vi "WPI_AccelerometerADXL362_SPI_Open.vi"(7 "SPI Bus":T1=enum."Invalid", 8 "error in":errorcluster, 9 "Accel Range":T2 items=["+/- 2 g", "+/- 4 g", "+/- 8 g"], 10 "ADXL345 Axes":T3={"X-Axis"=TRUE, "Y-Axis"=FALSE, "Z-Axis"=FALSE}) -> (0 "error out":errorcluster, 3 "AccelerometerDevRef":T4={"DevStatus"={"status"=FALSE, "code"=0, "source"=""}, "Scaling"={"Gain (VoltsPerG)"=0.0, "Center Voltage"=0.0}, "Analog Channels"={"X-Axis"=enum."Invalid", "Y-Axis"=enum."Invalid", "Z-Axis"=enum."Invalid"}, "I2C Bus"=enum."Invalid", "SPI Bus"=enum."Invalid", "Accel Range"=0, "ADXL Axes"={"X-Axis"=FALSE, "Y-Axis"=FALSE, "Z-Axis"=FALSE}, "Handle"=0, "Device Address"=0, "Accel Type"=enum."Analog"} {"Device Address" format="%.0x"; "Accel Range" items=["+/- 2 g", "+/- 4 g", "+/- 8 g", "+/- 16 g"]})   [LabVIEW 2017]
doc: "Opens a reference to the accelerometer you specify. You must open a reference before using any other VIs on this palette.\n\nThis software is licensed. Open the labview\\readme\\WPI Robotics Library Open Source License.txt file for more information."
uses:
  <vilib>/Rock Robotics/WPI/Accelerometer/WPI_AccelerometerDevRef.ctl
  <vilib>/Rock Robotics/WPI/Accelerometer/WPI_AccelerometerScaling.ctl
  <vilib>/Rock Robotics/WPI/Accelerometer/WPI_AccelerometerAnalogChannels.ctl
  <vilib>/Rock Robotics/SystemInterfaces/AI/FPGA_AIChannel.ctl
  <vilib>/Rock Robotics/SystemInterfaces/i2clib/i2c_bus.ctl
  <vilib>/Rock Robotics/SystemInterfaces/spilib/spi_bus.ctl
  <vilib>/Rock Robotics/WPI/Accelerometer/ADXL345 Range.ctl
  <vilib>/Rock Robotics/WPI/Accelerometer/WPI_AccelerometerADXL345 Axes.ctl
  <vilib>/Rock Robotics/WPI/Accelerometer/ADXL362 Range.ctl
  <vilib>/Rock Robotics/SystemInterfaces/NetworkCommunication/NetComm_UsageReport_ResourceType.ctl
  <vilib>/Rock Robotics/WPI/SPI/WPI_SPIMode.ctl
panel:
  # "ADXL"
  # "Analog"
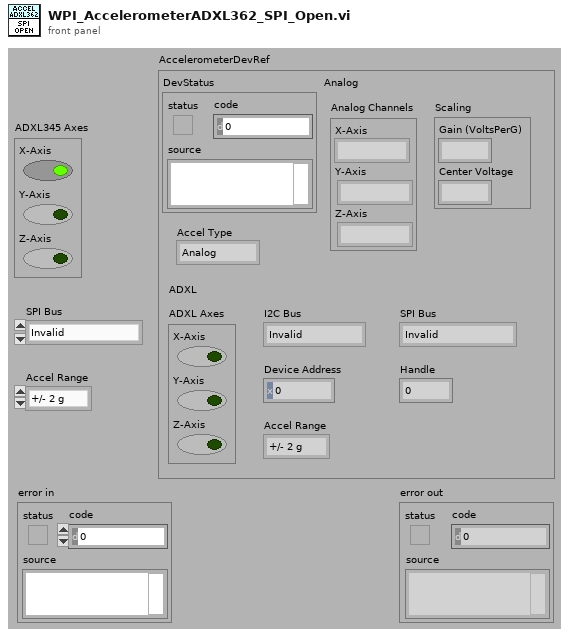
[diagram p1: front panel]
types:
  T1 = typedef "spi_bus.ctl" = enum16{"SPI On-Board, CS0", "SPI On-Board, CS1", "SPI On-Board, CS2", "SPI On-Board, CS3", "SPI MXP", "Invalid"}
  T2 = typedef "ADXL362 Range.ctl" = u8
  T3 = typedef "WPI_AccelerometerADXL345 Axes.ctl" = cluster{"X-Axis":bool, "Y-Axis":bool, "Z-Axis":bool}
  T4 = typedef "WPI_AccelerometerDevRef.ctl" = cluster{"DevStatus":errorcluster, "Scaling":T5, "Analog Channels":T6, "I2C Bus":T8, "SPI Bus":T1, "Accel Range":T9, "ADXL Axes":T3, "Handle":i32, "Device Address":u8, "Accel Type":enum16{"Analog", "ADXL345 I2C", "ADXL345 SPI", "Internal", "ADXL362 SPI"}}
  T5 = typedef "WPI_AccelerometerScaling.ctl" = cluster{"Gain (VoltsPerG)":dbl, "Center Voltage":dbl}
  T6 = typedef "WPI_AccelerometerAnalogChannels.ctl" = cluster{"X-Axis":T7, "Y-Axis":T7, "Z-Axis":T7}
  T7 = typedef "FPGA_AIChannel.ctl" = enum8{"AI 0", "AI 1", "AI 2", "AI 3", "AI MXP 0", "AI MXP 1", "AI MXP 2", "AI MXP 3", "Invalid"}
  T8 = typedef "i2c_bus.ctl" = enum16{"I2C On-Board", "I2C MXP", "Invalid"}
  T9 = typedef "ADXL345 Range.ctl" = u8
  T10 = typedef "WPI_SPIMode.ctl" = enum16{"Mode 0 (Clk Idle Low,Sample on Leading)", "Mode 1 (Clk Idle Low,Sample on Trailing)", "Mode 2 (Clk Idle High,Sample on Leading)", "Mode 3 (Clk Idle High,Sample on Trailing)"}
  T11 = typedef "NetComm_UsageReport_ResourceType.ctl" = enum8{"Controller", "Module", "Language", "CANPlugin", "Accelerometer", "ADXL345", "AnalogChannel", "AnalogTrigger", "AnalogTriggerOutput", "CANJaguar", "Compressor", "Counter", "Dashboard", "DigitalInput", "DigitalOutput", "DriverStationCIO", "DriverStationEIO", "DriverStationLCD", "Encoder", "GearTooth", "Gyro", "I2C", "Framework", "Jaguar", "Joystick", "Kinect", "KinectStick", "PIDController", "Preferences", "PWM", "Relay", "RobotDrive", "SerialPort", "Servo", "Solenoid", "SPI", "Task", "Ultrasonic", "Victor", "Button", "Command", "AxisCamera", "PCVideoServer", "SmartDashboard", "Talon", "HiTechnicColorSensor", "HiTechnicAccel", "HiTechnicCompass", "SRF08", "AnalogOutput", "Victor SP", "Talon SRX", "CAN Talon SRX", "ADXL362 Accel", "ADXRS450 Gyro", "Rev SPARK", "Mindsensors SD540", "Digital Filter", "ADIS16448", "PDP", "PCM", "PigeonIMU", "Nidec Brushless", "CTRE CANifier", "CTRE Future 0", "CTRE Future 1", "CTRE Future 2", "CTRE Future 3", "CTRE Future 4", "CTRE Future 5", "CTRE Future 6"}
  T12 = typedef "WPI_SPIDevRef.ctl" = cluster{"DevStatus":errorcluster, "Handle":i32, "SPI Bus":T1}
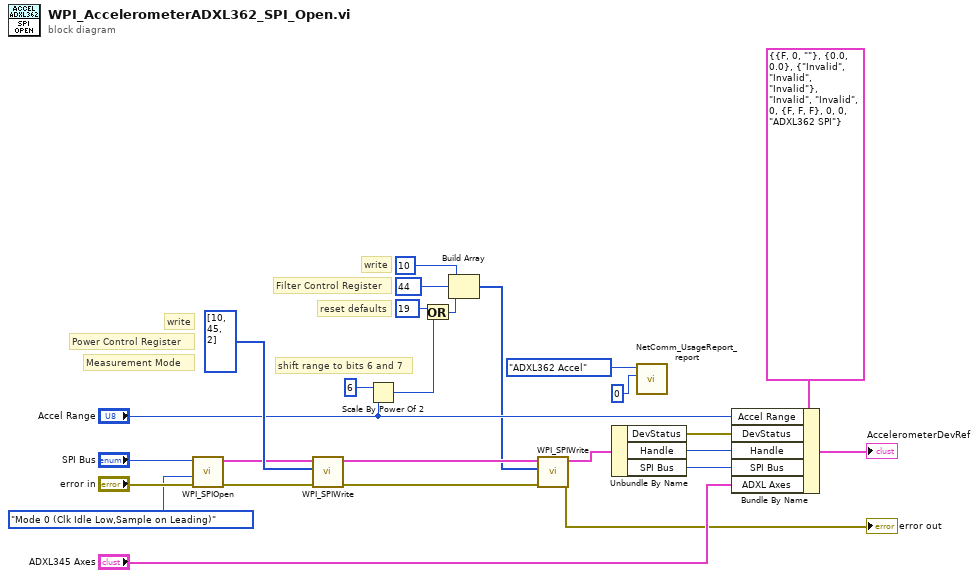
[diagram p0: block diagram]
diagram:
  # "shift range to bits 6 and 7"
  # "reset defaults"
  # "Filter Control Register"
  # "write"
  # "Measurement Mode"
  # "Power Control Register"
  # "write"
  n1 = call <vilib>:"WPI_SPIOpen.vi"("error in"="error in", "Mode (3)"=WPI_SPIMode."Mode 0 (Clk Idle Low,Sample on Leading)", "SPI Bus"="SPI Bus") -> ("error out"=w19:errorcluster, "SPIDevRef"=w17:T12)  [unwired: 3 in, 4 out]
  n2 = call <vilib>:"WPI_SPIWrite.vi"("error in (no error)"=w19, "Data To Send"=u8[] [10, 45, 2], "SPIDevRef"=w17) -> ("error out"=w20:errorcluster, "SPIDevRef"=w16:T12)  [unwired: 7 out]
  n3 = Scale By Power Of 2(n=i16 6, x="Accel Range") -> (x*2^n=w4:T2)
  n4 = Or(x=u8 19 ("Data To Send"), y=w4) -> (x .or. y?=w3:T2)
  n5 = Build Array(u8 10 ("Data To Send"), u8 44 ("Data To Send"), w3) -> (w6:T2[])
  n6 = call <vilib>:"WPI_SPIWrite.vi"("error in (no error)"=w20, "Data To Send"=w6, "SPIDevRef"=w16) -> ("error out"=→"error out":errorcluster, "SPIDevRef"=w5:T12)  [unwired: 7 out]
  n7 = Unbundle By Name(w5) -> ("DevStatus"=w24:errorcluster, "Handle"=w22:i32, "SPI Bus"=w23:T1)
  n8 = call <vilib>:"NetComm_UsageReport_report.vi"("Instance Number"=u8 0, "Resource Type"=NetComm_UsageReport_ResourceType."ADXL362 Accel") -> ()  [unwired: 10 in]
  n9 = Bundle By Name(cluster=T4 {"DevStatus"={"status"=FALSE, "code"=0, "source"=""}, "Scaling"={"Gain (VoltsPerG)"=0.0, "Center Voltage"=0.0}, "Analog Channels"={"X-Axis"=enum."Invalid", "Y-Axis"=enum."Invalid", "Z-Axis"=enum."Invalid"}, "I2C Bus"=enum."Invalid", "SPI Bus"=enum."Invalid", "Accel Range"=0, "ADXL Axes"={"X-Axis"=FALSE, "Y-Axis"=FALSE, "Z-Axis"=FALSE}, "Handle"=0, "Device Address"=0, "Accel Type"=enum."ADXL362 SPI"} ("AccelerometerDevRef"), "Accel Range"="Accel Range", "DevStatus"=w24, "Handle"=w22, "SPI Bus"=w23, "ADXL Axes"="ADXL345 Axes") -> (→"AccelerometerDevRef":T4)
